vi "meetCriteria.vi"(8 "error in (no error)":errorcluster, 10 "Persons In":refnum<class "Person.lvclass">[](array[class]), 11 "CiteriaSingle in":refnum<class "CiteriaSingle.lvclass">) -> (0 "error out":errorcluster, 2 "Persons Out":refnum<class "Person.lvclass">[](array[class]), 3 "CiteriaSingle out":refnum<class "CiteriaSingle.lvclass">)   [LabVIEW 2017, in "CiteriaSingle.lvclass"]
uses:
  CiteriaSingle.lvclass
  Person Class/Person.lvclass
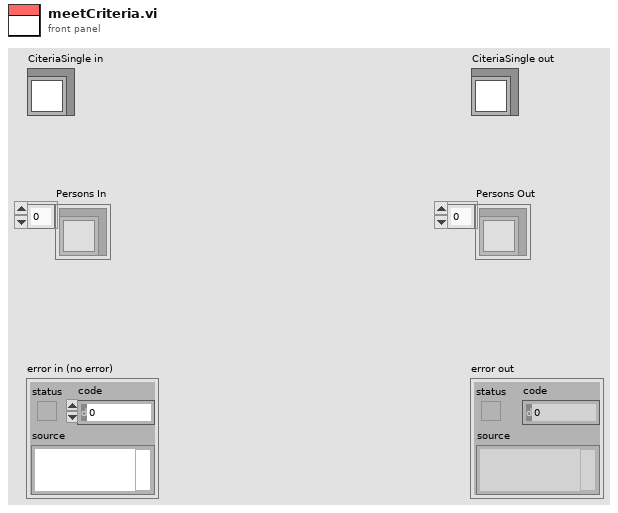
[diagram p1: front panel]
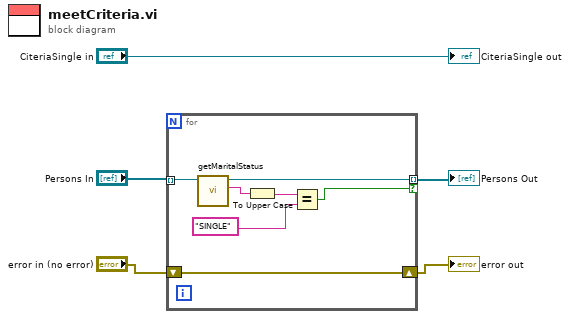
[diagram p0: block diagram]
diagram:
  n1 = for {
    shift-right: [w12] -> w3
    shift-left: "error in (no error)" -> [w12]
    tunnel: "Persons In" -> [w11] mode=indexing
    tunnel: [w7] -> w2 mode=indexing if=w6
    n2 = call-dynamic "getMaritalStatus.vi"("Person in"=w11) -> ("maritalStatus"=w10:string, "Person out"=w7:refnum<class "Person.lvclass">)  [unwired: 8 in, 1 out]
    n3 = To Upper Case(1:w10) -> (0:w9:string)
    n4 = Equal?(x=w9, y="SINGLE") -> (x = y?=w6:bool)
  }
  "error out" <- w3
  "Persons Out" <- w2
  "CiteriaSingle out" <- "CiteriaSingle in"
